vi "test.VariantWrapper.vi"() -> ()   [LabVIEW 2014]
uses:
  Private/Class/meth.Constructor.vi
  Private/Class/meth.Destructor.vi
  GLue.lvlib
panel:
  out "error out":errorcluster
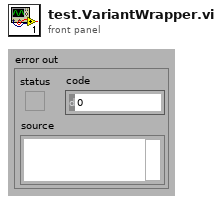
[diagram p1: front panel]
types:
  T1 = cluster{"int":i32, "string":string, "This VI":refnum<vi>}
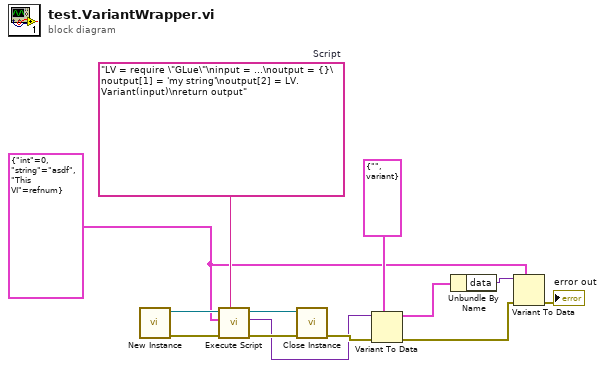
[diagram p0: block diagram]
diagram:
  w2 = T1 {"int"=0, "string"="asdf", "This VI"=refnum}
  w9 = "LV = require \"GLue\"\ninput = ...\noutput = {}\noutput[1] = 'my string'\noutput[2] = LV.Variant(input)\nreturn output"  # Script
  n1 = call "New Instance.vi"() -> ("error out"=w13:errorcluster, "GLue out"=w12:refnum<class "class.GLue.lvclass">)  [unwired: 10 in]
  n2 = call "Execute Script.vi"("Script"=w9, "error in"=w13, "Argument Data"=w2, "GLue in"=w12) -> ("error out"=w11:errorcluster, "Return Data"=w7:variant, "GLue out"=w10:refnum<class "class.GLue.lvclass">)  [unwired: 5 in]
  n3 = call "Close Instance.vi"("error in"=w11, "GLue in"=w10) -> ("error out"=w8:errorcluster)  [unwired: 9 in]
  n4 = Variant To Data(error in=w8, type=cluster{"string":string, "data":variant} {"string"="", "data"=variant}, Variant=w7) -> (data=w5:cluster{"string":string, "data":variant}, error out=w3:errorcluster)
  n5 = Unbundle By Name(w5) -> ("data"=w4:variant)
  n6 = Variant To Data(error in=w3, type=w2, Variant=w4) -> (error out=→"error out":errorcluster)  [unwired: 1 out]
